vi "Cal Inst - Take Electrical Measurements.vi"(8 "error in (no error)":errorcluster, 9 "UI":refnum<queue>, 10 "Temperature in":dbl, 11 "VISA Refnum in":refnum<visa-resource-name>) -> (0 "error out":errorcluster, 2 "Electrical Data 2":T1, 3 "VISA Refnum out":refnum<visa-resource-name>)   [LabVIEW 2013]
uses:
  controls/electrical2.ctl
  support/Message Queue/Message Cluster.ctl
  support/Message Queue/Cal Inst Message Queue.lvlib
  Cal Inst Acquisition.lvlib
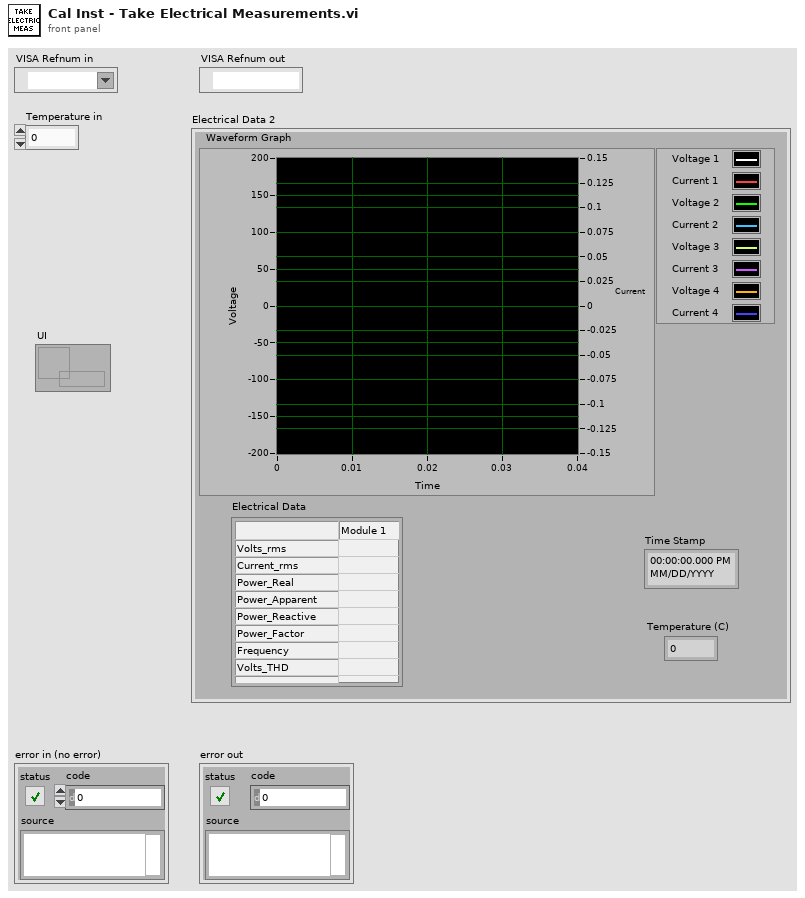
[diagram p1: front panel]
types:
  T1 = typedef "Cal Inst.lvlib/Cal Inst Acquisition.lvlib/electrical2.ctl" = cluster{"Time Stamp":timestamp, "Temperature (C)":dbl, "Electrical Data":string[][], "Waveform Graph":waveform(dbl)[]}
  T2 = cluster{"seconds since 1Jan1904":timestamp, "Temperature in":dbl, string[][], "Waveform Graph":waveform(sgl)[]}
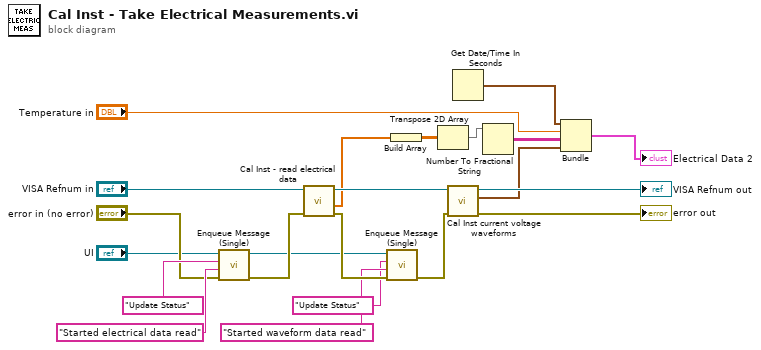
[diagram p0: block diagram]
diagram:
  n1 = call "Enqueue Message (Single).vi"("error in (no error)"="error in (no error)", "Message Data"="Started electrical data read" ("Message"), "Message"="Update Status", "Message Queue"="UI") -> ("error out"=w9:errorcluster, "dup Message Queue"=w5:refnum<queue>)  [unwired: 6 in]
  n2 = call "Cal Inst - read electrical data.vi"("error in (no error)"=w9, "VISA Refnum in"="VISA Refnum in") -> ("error out"=w7:errorcluster, "Electrical Data"=w18:dbl[], "VISA Refnum out"=w20:refnum<visa-resource-name>)  [unwired: 6 in, 1 out]
  n3 = call "Enqueue Message (Single).vi"("error in (no error)"=w7, "Message Data"="Started waveform data read" ("Message"), "Message"="Update Status", "Message Queue"=w5) -> ("error out"=w6:errorcluster)  [unwired: 6 in, 1 out]
  n4 = Build Array(w18) -> (w2:dbl[][])
  n5 = Transpose 2D Array(2D array=w2) -> (transposed array=w1:dbl[][])
  n6 = call "Cal Inst current voltage waveforms.vi"("error in (no error)"=w6, "VISA resource name"=w20) -> ("error out"=→"error out":errorcluster, "Waveform Graph"=w13:waveform(sgl)[], "VISA resource name out"=→"VISA Refnum out":refnum<visa-resource-name>)  [unwired: 7 in]
  n7 = Get Date/Time In Seconds() -> (seconds since 1Jan1904=w17:timestamp)
  n8 = Number To Fractional String(number=w1) -> (F-format string=w14:string[][])  [unwired: 3 in]
  n9 = Bundle("seconds since 1Jan1904"=w17, "Temperature in"="Temperature in", w14, "Waveform Graph"=w13) -> (→"Electrical Data 2":T2)  [unwired: 1 in]
